vi "LoadStepType.vi"(8 "error in (no error)":errorcluster, 9 "Step Class Library":T1, 10 "Step Type":string, 11 "StepNode in":refnum<class "StepNode.lvclass">) -> (0 "error out":errorcluster, 3 "StepNode out":refnum<class "StepNode.lvclass">)   [LabVIEW 2015, in "StepNode.lvclass"]
uses:
  StepNode.lvclass
  Controls/StepClassLibrary.ctl
  Prototype/classes/Step/Config/Step Config.lvclass
  Prototype/classes/Step/UI/Step UI.lvclass
  <vilib>/Utility/error.llb/Error Cluster From Error Code.vi
  <vilib>/ErrorRing/Error Ring.xnode
  Configuration Tool.lvlib
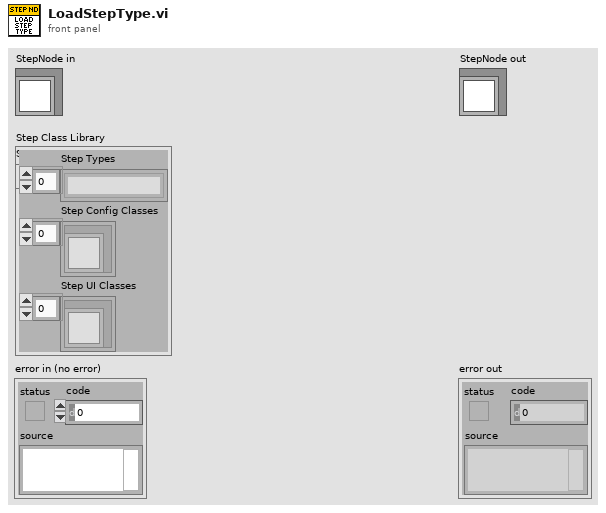
[diagram p1: front panel]
types:
  T1 = typedef "Configuration Tool.lvlib/StepClassLibrary.ctl" = cluster{"Step Types":string[], "Step Config Classes":refnum<class "Step Config.lvclass">[], "Step UI Classes":refnum<class "Step UI.lvclass">[]}
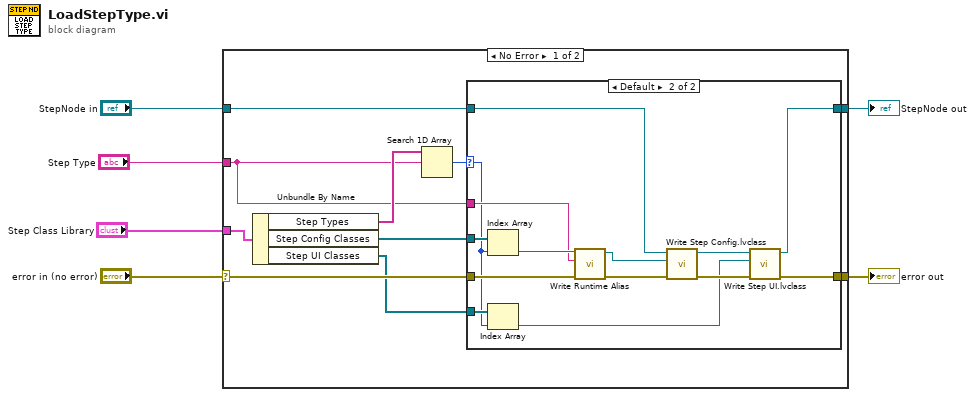
[diagram p0: block diagram]
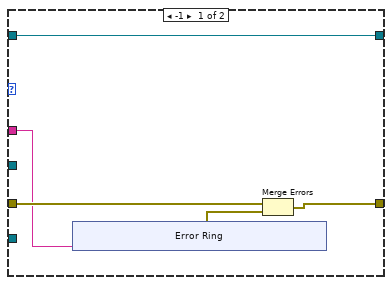
[diagram p2: hidden frame]
diagram:
  n1 = case shown="No Error" "error in (no error)" {
    selector: "error in (no error)" -> [w10 w44]
    tunnel: [w9 w44] -> w5
    tunnel: [w14 w43] -> w3
    tunnel: "StepNode in" -> [w16 w43]
    tunnel: "Step Class Library" -> [w15 _]
    tunnel: "Step Type" -> [w8 _]
    frame No Error {
      n2 = Unbundle By Name(w15) -> ("Step Types"=w12:string[], "Step Config Classes"=w13:refnum<class "Step Config.lvclass">[], "Step UI Classes"=w7:refnum<class "Step UI.lvclass">[])
      n3 = Search 1D Array(1D array=w12, element=w8) -> (index of element=w11:i32)  [unwired: 1 in]
      n4 = case shown="Default" w11 {
        selector: w11 -> [_ w30]
        tunnel: w16 -> [w21 w42]
        tunnel: [w21 w32] -> w14
        tunnel: w13 -> [_ w41]
        tunnel: w10 -> [w20 w40]
        tunnel: [w19 w34] -> w9
        tunnel: w8 -> [w17 w35]
        tunnel: w7 -> [_ w31]
        frame -1 {
          n5 = xnode "Error Ring"("parameter 0"=w17) -> ("error out"=w18:errorcluster)
          n6 = Merge Errors(w20, w18) -> (w19:errorcluster)
        }
        frame Default {
          n7 = Index Array(array=w41, index=w30) -> (element=w37:refnum<class "Step Config.lvclass">)
          n8 = Index Array(array=w31, index=w30) -> (element=w29:refnum<class "Step UI.lvclass">)
          n9 = call-dynamic "Write Runtime Alias.vi"("error in (no error)"=w40, "Runtime Alias"=w35, "Step Config in"=w37) -> ("error out"=w38:errorcluster, "Step Config out"=w36:refnum<class "Step Config.lvclass">)  [unwired: 7 in]
          n10 = call-dynamic "Write Step Config.lvclass.vi"("error in (no error)"=w38, "Step Config.lvclass"=w36, "StepNode in"=w42) -> ("error out"=w39:errorcluster, "StepNode out"=w33:refnum<class "StepNode.lvclass">)  [unwired: 7 in]
          n11 = call-dynamic "Write Step UI.lvclass.vi"("error in (no error)"=w39, "Step UI.lvclass"=w29, "StepNode in"=w33) -> ("error out"=w34:errorcluster, "StepNode out"=w32:refnum<class "StepNode.lvclass">)  [unwired: 7 in]
        }
      }
    }
    frame Error {
    }
  }
  "error out" <- w5
  "StepNode out" <- w3
